vi "To JSON Tree.vi"(8 "error in (no error)":errorcluster, 11 "Response in":refnum<class "Response.lvclass">) -> (0 "error out":errorcluster, 2 "JSON out":refnum<class "JSON Null.lvclass">, 3 "Response out":refnum<class "Response.lvclass">)   [LabVIEW 2015, in "Response.lvclass"]
uses:
  Response.lvclass
  <vilib>/NI/JSON Support for LabVIEW/JSON Data Classes/JSON Datatype/JSON Null.lvclass
  Response.lvclass/Response.ctl
  Has ID.vi
  <vilib>/NI/JSON Support for LabVIEW/JSON Data Classes/JSON Object/New JSON Object (Empty).vi
  <vilib>/NI/JSON Support for LabVIEW/JSON Data Classes/JSON Object/Insert Key Value Pair (Single String).vi
  <vilib>/NI/JSON Support for LabVIEW/JSON Data Classes/JSON Object/Insert Key Value Pair (Single).vi
  error/error.lvclass
  New folder/result.lvclass
  id/id.lvclass
  <vilib>/NI/JSON Support for LabVIEW/JSON Data Classes/JSON Helper/JSON Helper.lvclass
  <vilib>/NI/JSON Support for LabVIEW/JSON Data Classes/JSON Object/JSON Object.lvclass
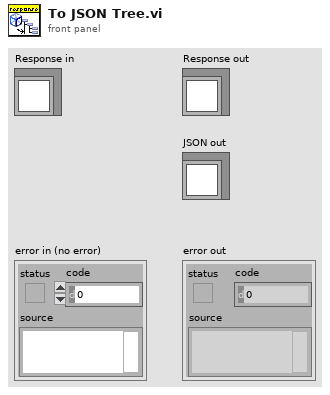
[diagram p1: front panel]
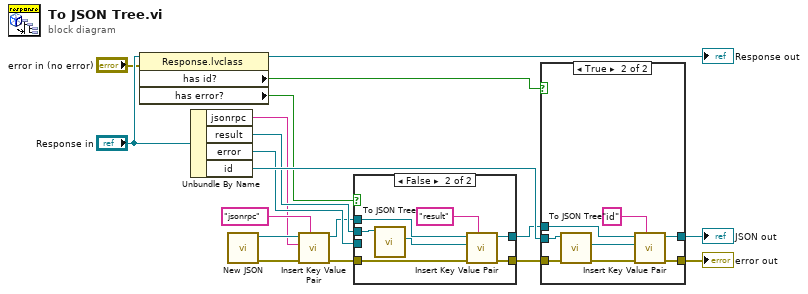
[diagram p0: block diagram]
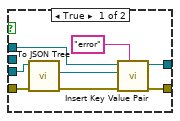
[diagram p2: hidden frame]
diagram:
  n1 = property class="Response.lvclass"(reference="Response in", error in="error in (no error)") -> (reference out=→"Response out":refnum<class "Response.lvclass">, "has id?"=w17:bool, "has error?"=w12:bool)  [unwired: 1 out]
  n2 = Unbundle By Name("Response in") -> ("jsonrpc"=w7:string, "result"=w14:refnum<class "result.lvclass">, "error"=w13:refnum<class "error.lvclass">, "id"=w16:refnum<class "id.lvclass">)
  n3 = call-poly <vilib>:"New JSON.vi"() -> ("error out"=w9:errorcluster, "JSON Object out"=w10:refnum<class "JSON Object.lvclass">)  [unwired: 10 in]
  n4 = call-poly <vilib>:"Insert Key Value Pair.vi"("key"="jsonrpc" ("Name"), "error in (no error)"=w9, "value"=w7, "JSON Object in"=w10) -> ("error out"=w4:errorcluster, "JSON Object out"=w6:refnum<class "JSON Object.lvclass">)  [unwired: 5 in, 1 out]
  n5 = case shown="False" w12 {
    tunnel: w13 -> [w25 _]
    tunnel: w14 -> [_ w29]
    tunnel: w6 -> [w23 w31]
    tunnel: [w22 w30] -> w5
    tunnel: w4 -> [w21 w28]
    tunnel: [w19 w27] -> w3
    frame True {
      n6 = call-dynamic "To JSON Tree.vi"("error in (no error)"=w21, "error in"=w25) -> ("error out"=w20:errorcluster, "JSON out"=w24:refnum<class "JSON Null.lvclass">)  [unwired: 7 in, 1 out]
      n7 = call-poly <vilib>:"Insert Key Value Pair.vi"("key"="error", "error in (no error)"=w20, "value"=w24, "JSON Object in"=w23) -> ("error out"=w19:errorcluster, "JSON Object out"=w22:refnum<class "JSON Object.lvclass">)  [unwired: 5 in, 1 out]
    }
    frame False {
      n8 = call-dynamic "To JSON Tree.vi"("result in"=w29) -> ("JSON out"=w32:refnum<class "JSON Null.lvclass">)  [unwired: 8 in, 2 out]
      n9 = call-poly <vilib>:"Insert Key Value Pair.vi"("key"="result", "error in (no error)"=w28, "value"=w32, "JSON Object in"=w31) -> ("error out"=w27:errorcluster, "JSON Object out"=w30:refnum<class "JSON Object.lvclass">)  [unwired: 5 in, 1 out]
    }
  }
  n10 = case shown="True" w17 {
    tunnel: w16 -> [_ w43]
    tunnel: w5 -> [w34 w42]
    tunnel: w3 -> [w35 w39]
    tunnel: [w35 w37] -> w2
    tunnel: [w34 w36] -> w1
    frame False {
    }
    frame True {
      n11 = call-dynamic "To JSON Tree.vi"("error in (no error)"=w39, "id in"=w43) -> ("error out"=w38:errorcluster, "JSON out"=w41:refnum<class "JSON Null.lvclass">)  [unwired: 7 in, 1 out]
      n12 = call-poly <vilib>:"Insert Key Value Pair.vi"("key"="id" ("Name"), "error in (no error)"=w38, "value"=w41, "JSON Object in"=w42) -> ("error out"=w37:errorcluster, "JSON Object out"=w36:refnum<class "JSON Object.lvclass">)  [unwired: 5 in, 1 out]
    }
  }
  "error out" <- w2
  "JSON out" <- w1
